vi "Verify as Binary File.vi"(5 "Options":T1, 7 "Test VI (caller)":string, 8 "error in":errorcluster, 9 "Extension":string, 10 "Binary File to Verify":path) -> (0 "error out":errorcluster)   [LabVIEW 2020, in "Caraya.Extension.lvlib"]
uses:
  Caraya.Extension.lvlib
  <vilib>/addons/_JKI Toolkits/Caraya/classes/Assert/Assert True.vi
  <vilib>/addons/_JKI Toolkits/Caraya/classes/Assert/Assert.lvclass
  Approval Tests/Approval Tests.lvlib
  Approval Tests/Reporter/Reporter.lvclass
  Approval Tests/Printer/Printer.lvclass
  Approval Tests/Options.ctl
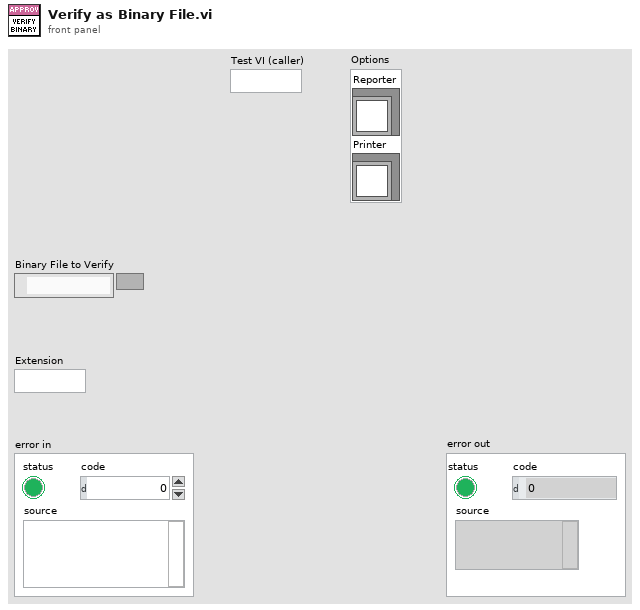
[diagram p1: front panel]
types:
  T1 = typedef "Approval Tests.lvlib/Options.ctl" = cluster{"Reporter":refnum<class "Reporter.lvclass">, "Printer":refnum<class "Printer.lvclass">}
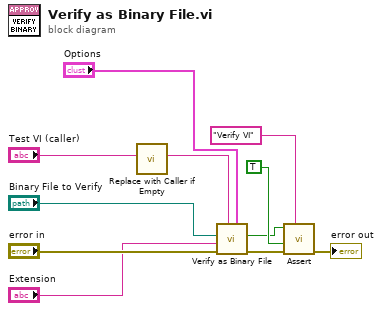
[diagram p0: block diagram]
diagram:
  n1 = call "Replace with Caller if Empty.vi"("Test VI (caller) in"="Test VI (caller)") -> ("Test VI (caller) out"=w3:string)  [unwired: 10 in]
  n2 = call "Verify as Binary File.vi"("Options"="Options", "Test VI (caller)"=w3, "error in"="error in", "Extension"="Extension", "Path to Binary File to Verify"="Binary File to Verify") -> ("error out"=w7:errorcluster, "Passed?"=w6:bool)  [unwired: 4 in, 1 out]
  n3 = call-poly <vilib>:"Assert.vi"("Label"="Verify VI", "error in (no error)"=w7, "Register with caller test (F)"=TRUE, "True?"=w6) -> ("error out"=→"error out":errorcluster)  [unwired: 6 in, 1 out]
